vi "filetest.vi"() -> ()   [LabVIEW 2017]
uses:
  <vilib>/Utility/config.llb/NI_LVConfig.lvlib
panel:
  out "size(s)":i32
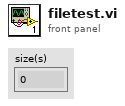
[diagram p1: front panel]
types:
  T1 = enum16{"open", "replace", "create", "open or create", "replace or create", "replace or create with confirmation"}
  T2 = typedef "NI_LVConfig.lvlib/Config Data RefNum.ctl" = refnum<k1>
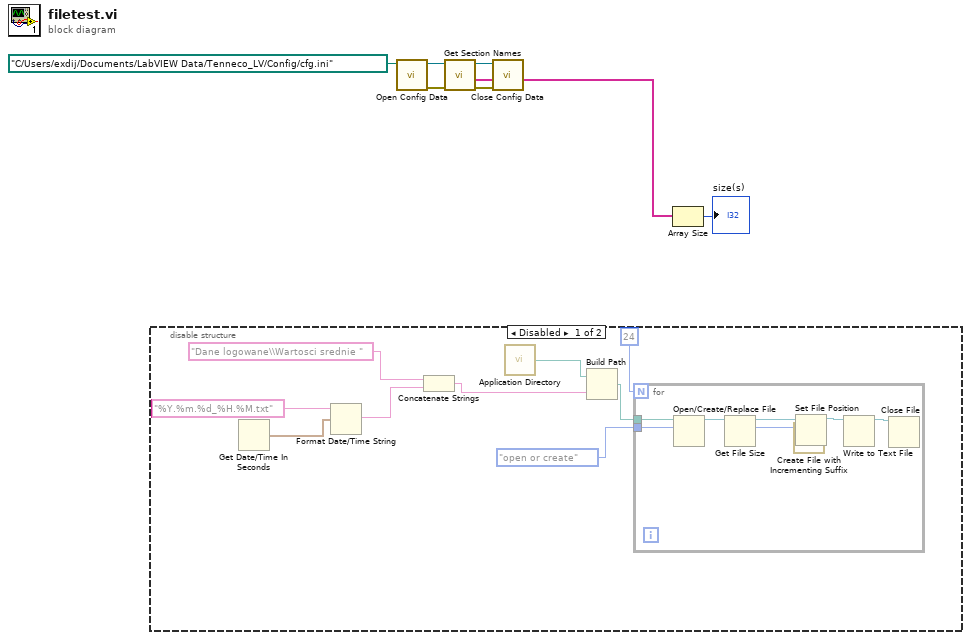
[diagram p0: block diagram]
diagram:
  n1 = disable-structure shown="Disabled" {
    frame Disabled {
      n2 = Get Date/Time In Seconds() -> (seconds since 1Jan1904=w12:timestamp)
      n3 = Format Date/Time String(time format string (%c)="%Y.%m.%d_%H.%M.txt", seconds (now)=w12) -> (date/time string=w13:string)  [unwired: 1 in]
      n4 = Concatenate Strings("Dane logowane\\Wartosci srednie " ("name or relative path"), w13) -> (w15:string)
      n5 = call <vilib>:"Application Directory.vi"() -> ("Application Directory"=w14:path)
      n6 = Build Path(base path=w14, name or relative path=w15) -> (appended path=w16:path)
      n7 = for {
        N: 24 -> [_]
        tunnel: w16 -> [w22]
        tunnel: T1."open or create" ("operation (0:open)") -> [w23]
        n8 = Open/Create/Replace File(file path (use dialog)=w22, operation (0:open)=w23) -> (refnum out=w21:refnum<file>)  [unwired: 4 in, 2 out]
        n9 = Get File Size(file=w21) -> (refnum out=w20:refnum<file>, size (in bytes)=w18:i64)  [unwired: 1 in, 1 out]
        n10 = Set File Position(offset (in bytes) (0)=w18, refnum=w20) -> (refnum out=w19:refnum<file>)  [unwired: 2 in, 1 out]
        n11 = Write to Text File(file (use dialog)=w19) -> (refnum out=w17:refnum<file>)  [unwired: 3 in, 2 out]
        n12 = Close File(refnum=w17) -> ()  [unwired: 1 in, 2 out]
      }
      n13 = call <vilib>:"Create File with Incrementing Suffix.vi"() -> ()  [unwired: 9 in, 3 out]
    }
    frame Enabled {
    }
  }
  n14 = call <vilib>:"Open Config Data.vi"("configuration file path"=path "C:/Users/exdij/Documents/LabVIEW Data/Tenneco_LV/Config/cfg.ini") -> ("error out"=w7:errorcluster, "refnum"=w6:T2)  [unwired: 8 in, 1 out]
  n15 = call <vilib>:"Get Section Names.vi"("error in (no error)"=w7, "refnum"=w6) -> ("error out"=w5:errorcluster, "section names"=w2:string[], "refnum out"=w4:T2)  [unwired: 7 in]
  n16 = call <vilib>:"Close Config Data.vi"("error in (no error)"=w5, "refnum"=w4) -> ()  [unwired: 8 in, 2 out]
  n17 = Array Size(array=w2) -> (size(s)=→"size(s)":i32)
